vi "camera stop - subvi.vi"   [LabVIEW 2014]
uses:
  Initilize Globals.vi
  lib/Andorlib/atmcd32d.dll
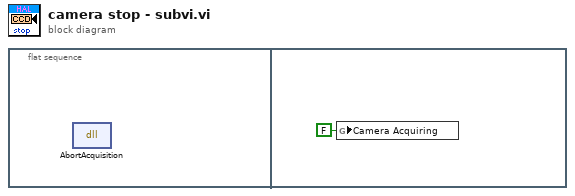
[diagram p0: block diagram]
diagram:
  n1 = flat-sequence {
    frame #0 {
      n2 = dll-call lib="C:/Users/Bakir/Desktop/LabFiles/Lambda2-Testing/lib/Andorlib/ATMCD32D.DLL" fn="AbortAcquisition" label="Call Library Function\nAbort"() -> ()  [unwired: 3 in, 3 out]
    }
    frame #1 {
      n3 = global write "Initilize Globals.vi" "Camera Acquiring"(FALSE ("Andor Aquiring")) -> ()
    }
  }
